vi "Close.vi"(8 "error in (no error)":errorcluster, 11 "Instrument.TC in":refnum<class "Instrument.TC.lvclass">) -> (0 "error out":errorcluster, 3 "Instrument.TC out":refnum<class "Instrument.TC.lvclass">)   [LabVIEW 2019, in "Instrument.TC.lvclass"]
uses:
  Instrument.TC.lvclass
  <userlib>/LevyLab/Instrument Framework/SMOs/Instrument/Instrument.lvclass
  C:/Program Files (x86)/National Instruments/LabVIEW 2019/user.lib/LevyLab/Instrument Framework/Instrument Types/Cryostat/Instrument.Cryostat.lvclass
  C:/Program Files (x86)/National Instruments/LabVIEW 2019/user.lib/LevyLab/Instrument Framework/SMOs/Instrument/Instrument.lvclass
  C:/Program Files (x86)/National Instruments/LabVIEW 2019/vi.lib/JKI/JKI SMO/SMO/SMO.lvclass
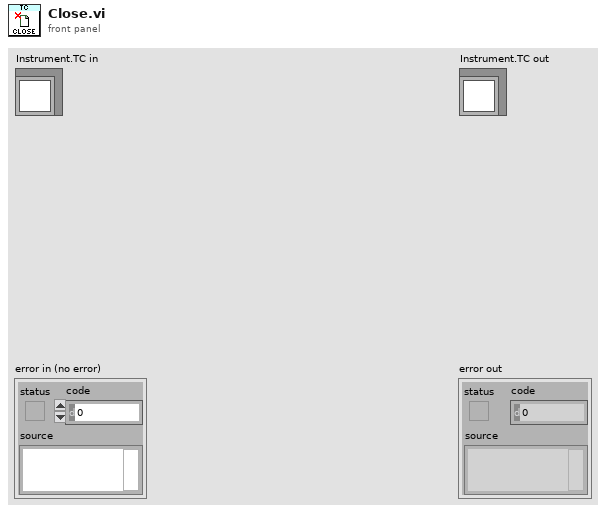
[diagram p1: front panel]
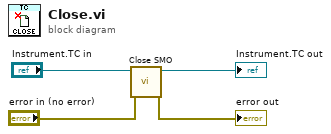
[diagram p0: block diagram]
diagram:
  n1 = call <userlib>:"Close SMO.vi"("error in (no error)"="error in (no error)", "Instrument in"="Instrument.TC in") -> ("error out"=→"error out":errorcluster, "Instrument out"=→"Instrument.TC out":refnum<class "Instrument.TC.lvclass">)  [unwired: 8 in]
